vi "Rasnik.vi"() -> ()   [LabVIEW 2015]
uses:
  GlobalPath.vi
  GlobalData.vi
panel:
  out "angle D10":dbl format="%.2f"
  out "angle D9":dbl format="%.2f"
  out "angle D8":dbl format="%.2f"
  out "angle D7":dbl format="%.2f"
  out "angle D6":dbl format="%.2f"
  out "angle D5":dbl format="%.2f"
  out "angle D4":dbl format="%.2f"
  out "angle D3":dbl format="%.2f"
  out "angle D2":dbl format="%.2f"
  out "angle D1":dbl format="%.2f"
  out "Y D10":dbl format="%.2f"
  out "Y D9":dbl format="%.2f"
  out "Y D8":dbl format="%.2f"
  out "Y D7":dbl format="%.2f"
  out "Y D6":dbl format="%.2f"
  out "Y D5":dbl format="%.2f"
  out "Y D4":dbl format="%.2f"
  out "Y D3":dbl format="%.2f"
  out "Y D2":dbl format="%.2f"
  out "Y D1":dbl format="%.2f"
  out "X D10":dbl format="%.2f"
  out "X D9":dbl format="%.2f"
  out "X D8":dbl format="%.2f"
  out "X D7":dbl format="%.2f"
  out "X D6":dbl format="%.2f"
  out "X D5":dbl format="%.2f"
  out "X D4":dbl format="%.2f"
  out "X D3":dbl format="%.2f"
  out "X D2":dbl format="%.2f"
  out "X D1":dbl format="%.2f"
  out "filenames 2":string[](array[string])
  out "Latest file: 2":path
  out "angle 6":string
  out "y 6":string
  out "x 6":string
  out "filenames":string[](array[string])
  out "path":path
  in  "Done?":bool
  out "angle 10":string
  out "y 10":string
  out "x 10":string
  out "angle 9":string
  out "y 9":string
  out "x 9":string
  out "angle 8":string
  out "y 8":string
  out "x 8":string
  out "angle 7":string
  out "y 7":string
  out "x 7":string
  out "angle 5":string
  out "y 5":string
  out "x 5":string
  out "angle 4":string
  out "y 4":string
  out "x 4":string
  out "angle 3":string
  out "y 3":string
  out "x 3":string
  out "angle 2":string
  out "y 2":string
  out "x 2":string
  out "angle 1":string
  out "y 1":string
  out "x 1":string
  out "Lines":string[](array[string])
  out "Latest file:":path
  in  "Open Program":bool
  in  "c-ccd 3":bool caption="Setup the electronics for the C-CCD reading"
  in  "c-ccd":bool caption="Read the data file"
  # "Rasmask reading from PCBs on stiffback/table"
  # "Run the C-CCD reading program \n(the 10 Rasmasks are automatically read and the data saved)"
  # "Data file reading"
  # "The most recent data file created by the C-CCD program will be opened.\nOnce the \"read data file\" is clicked, the raw data and displacement should appear on the PCB schematics on the bottom."
  # "Displacement (um):"
  # "Raw Data (um):"
  # "Rasmask 1"
  # "Rasmask 2"
  # "Rasmask 1"
  # "Rasmask 2"
  # "Rasmask 3"
  # "Rasmask 4"
  # "Rasmask 3"
  # "Rasmask 4"
  # "Rasmask 6"
  # "Rasmask 5"
  # "Rasmask 6"
  # "Rasmask 5"
  # "Rasmask 7"
  # "Rasmask 8"
  # "Rasmask 7"
  # "Rasmask 8"
  # "Rasmask 9"
  # "Rasmask 10"
  # "Rasmask 9"
  # "Rasmask 10"
  # "Open the DB and load the Rarnik raw file:\nClick on the tab \"RO measurement\" and on the bottom click on \"Load Rasnik 1\" for the table and \"Load  Rasnik 2\" for the stiffback\nLoad the file that appears here --------------------------------------------------------------->\nPress \"SAve info to database\""
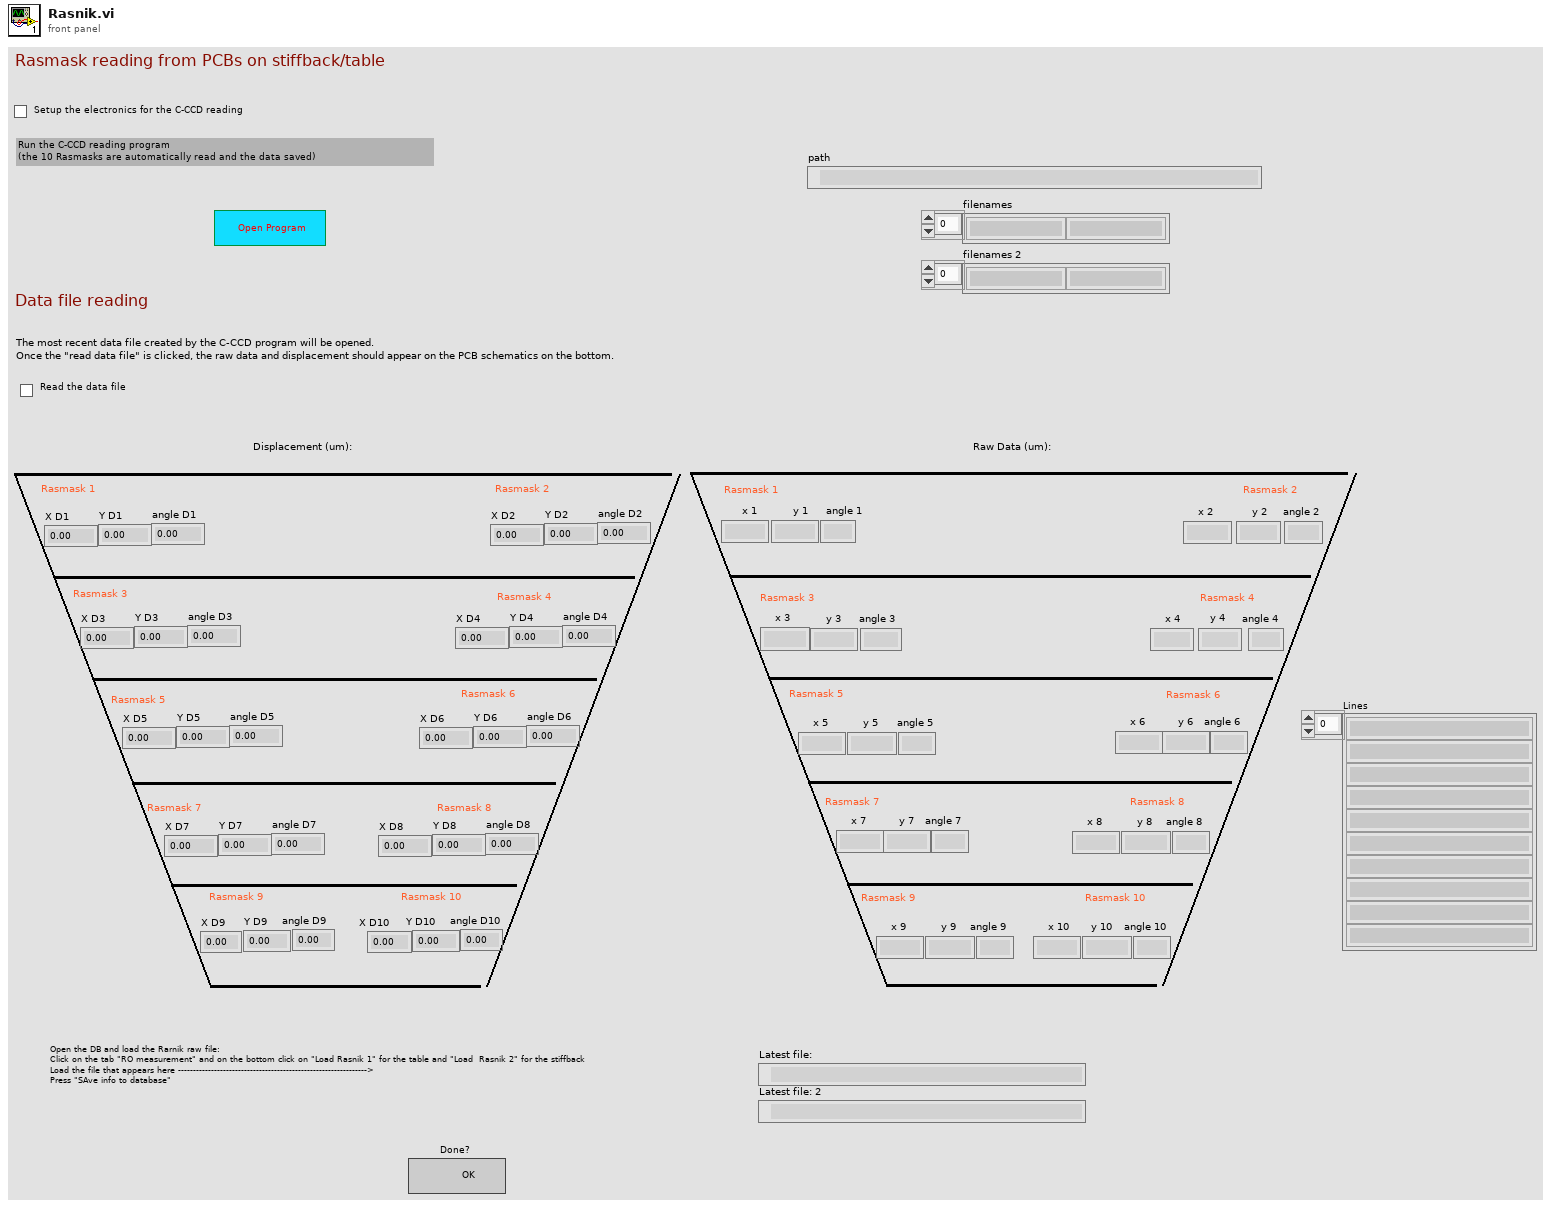
[diagram p1: front panel]
types:
  T1 = enum16{"open", "replace", "create", "open or create", "replace or create", "replace or create with confirmation"}
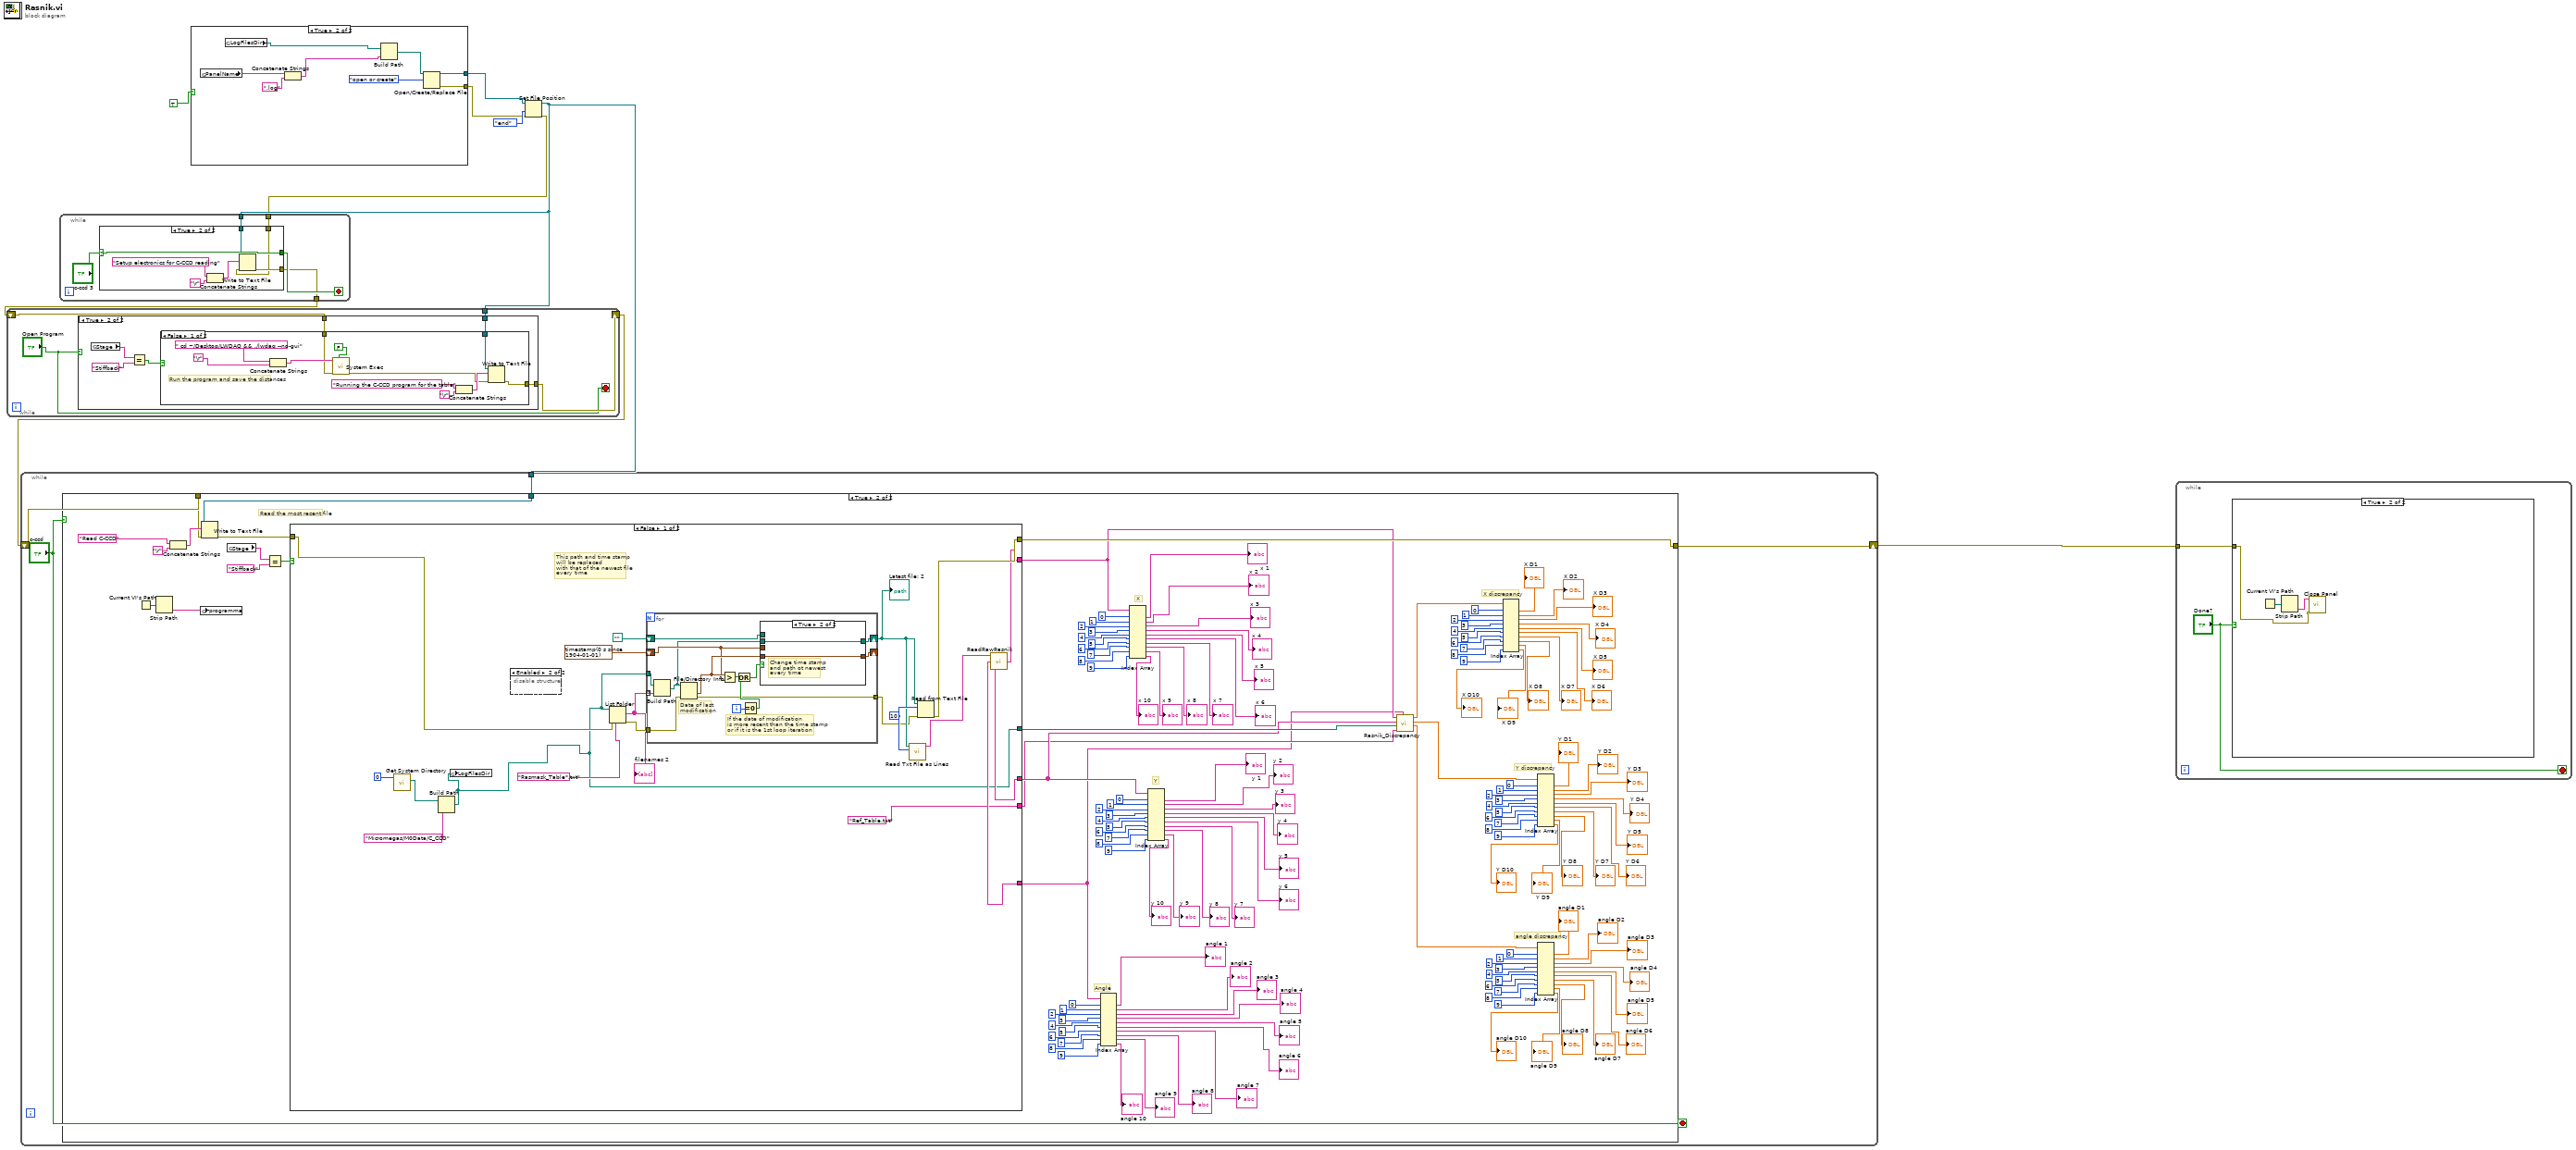
[diagram p0: block diagram]
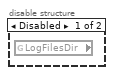
[diagram p4: hidden frame]
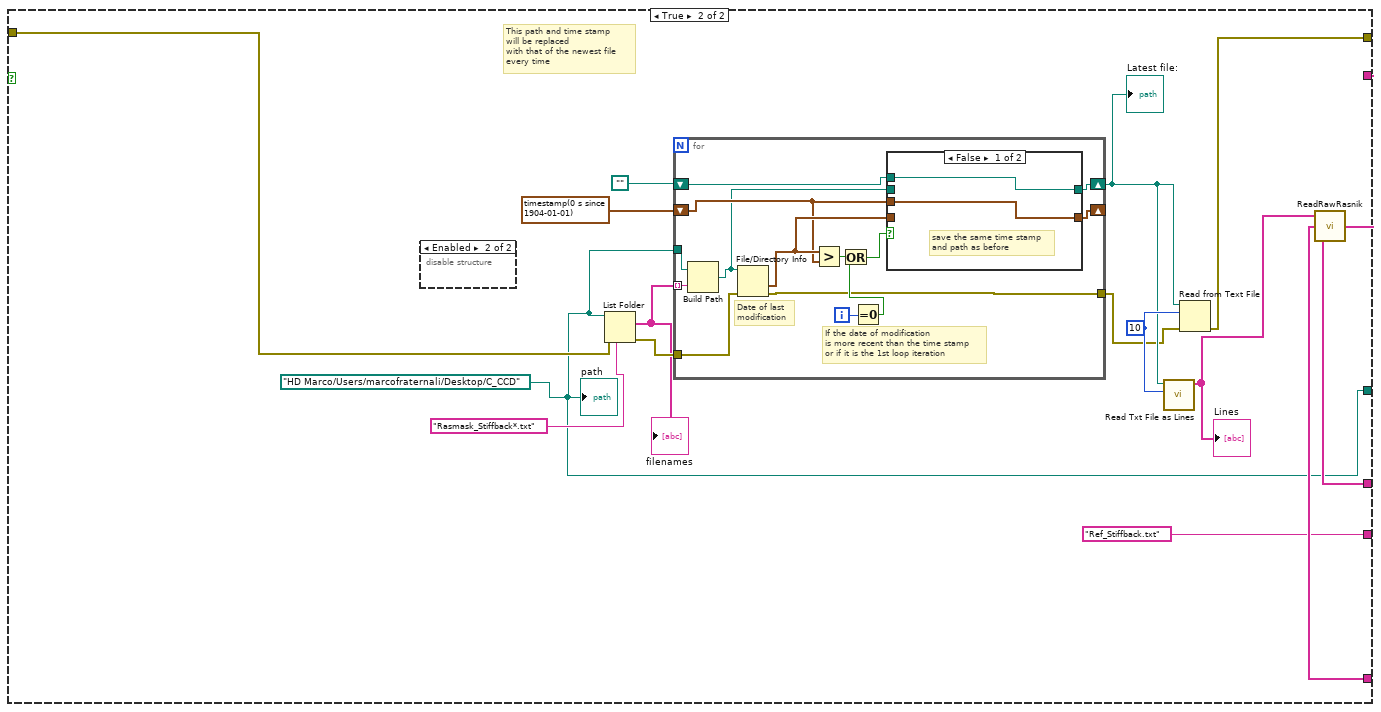
[diagram p6: hidden frame]
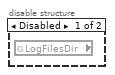
[diagram p7: hidden frame]
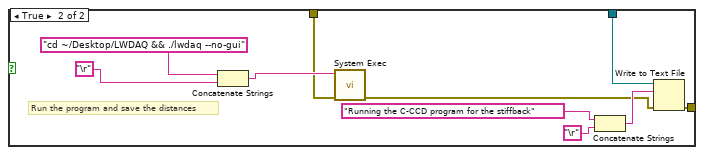
[diagram p11: hidden frame]
diagram:
  n1 = case shown="True" TRUE {
    tunnel: [_ w16] -> w3
    tunnel: [_ w15] -> w4
    frame False {
    }
    frame True {
      n2 = global read "GlobalData.vi" "PanelName"() -> (w11:string)
      n3 = global read "GlobalPath.vi" "LogFilesDir"() -> (w13:path)
      n4 = Concatenate Strings(w11, ".log") -> (w10:string)
      n5 = Build Path(base path=w13, name or relative path=w10) -> (appended path=w17:path)
      n6 = Open/Create/Replace File(file path (use dialog)=w17, operation (0:open)=T1."open or create") -> (refnum out=w16:refnum<file>, error out=w15:errorcluster)  [unwired: 4 in, 1 out]
    }
  }
  n7 = Set File Position(refnum=w3, from (0:start)=enum16{"start", "end", "current"}."end", error in=w4) -> (refnum out=w2:refnum<file>, error out=w1:errorcluster)  [unwired: 1 in]
  n8 = while {
    tunnel: w2 -> [w21]
    tunnel: [w19] -> w7
    tunnel: w1 -> [w18]
    stop <- w20 stop-if-true
    n9 = case shown="True" "c-ccd 3" {
      selector: "c-ccd 3" -> [_ w25]
      tunnel: [_ w26] -> w19
      tunnel: w21 -> [_ w23]
      tunnel: [_ w25] -> w20
      tunnel: w18 -> [_ w24]
      frame False {
      }
      frame True {
        n10 = Concatenate Strings("Setup electronics for C-CCD reading", "\r") -> (w29:string)
        n11 = Write to Text File(file (use dialog)=w23, text=w29, error in=w24) -> (error out=w26:errorcluster)  [unwired: 1 in, 2 out]
      }
    }
  }
  n12 = while {
    tunnel: w2 -> [w31]
    shift-right: [w32] -> w9
    shift-left: w7 -> [w33]
    stop <- "Open Program" stop-if-true
    n13 = case shown="True" "Open Program" {
      tunnel: w33 -> [w34 w37]
      tunnel: [w34 w36] -> w32
      tunnel: w31 -> [_ w35]
      frame False {
      }
      frame True {
        n14 = global read "GlobalData.vi" "Stage"() -> (w39:string)
        n15 = Equal?(x=w39, y="Stiffback") -> (x = y?=w38:bool)
        n16 = case shown="False" w38 {
          tunnel: w37 -> [w45 w55]
          tunnel: [w43 w53] -> w36
          tunnel: w35 -> [w42 w52]
          frame False {
            # "Run the program and save the distances"
            n17 = Concatenate Strings(" cd ~/Desktop/LWDAQ && ./lwdaq --no-gui", "\r") -> (w50:string)
            n18 = call <vilib>:"System Exec.vi"("wait until completion? (T)"=FALSE, "error in (no error)"=w45, "command line"=w50) -> ("error out"=w44:errorcluster)  [unwired: 5 in, 3 out]
            n19 = Concatenate Strings("Running the C-CCD program for the table", "\r") -> (w48:string)
            n20 = Write to Text File(file (use dialog)=w42, text=w48, error in=w44) -> (error out=w43:errorcluster)  [unwired: 1 in, 2 out]
          }
          frame True {
            # "Run the program and save the distances"
            n21 = Concatenate Strings("cd ~/Desktop/LWDAQ && ./lwdaq --no-gui", "\r") -> (w60:string)
            n22 = call <vilib>:"System Exec.vi"("error in (no error)"=w55, "command line"=w60) -> ("error out"=w54:errorcluster)  [unwired: 6 in, 3 out]
            n23 = Concatenate Strings("Running the C-CCD program for the stiffback", "\r") -> (w58:string)
            n24 = Write to Text File(file (use dialog)=w52, text=w58, error in=w54) -> (error out=w53:errorcluster)  [unwired: 1 in, 2 out]
          }
        }
      }
    }
  }
  n25 = while {
    tunnel: w2 -> [w63]
    shift-right: [w64] -> w8
    shift-left: w9 -> [w65]
    stop <- "c-ccd" stop-if-true
    n26 = case shown="True" "c-ccd" {
      tunnel: w65 -> [w66 w198]
      tunnel: [w66 w196] -> w64
      tunnel: w63 -> [_ w195]
      frame False {
      }
      frame True {
        # "angle discrepancy"
        # "Y discrepancy"
        # "X discrepancy"
        # "Angle"
        # "Y"
        # "X"
        # "Read the most recent file"
        n27 = Current VI's Path() -> (path=w199:path)
        n28 = Strip Path(path=w199) -> (name=w200:string)  [unwired: 1 out]
        n29 = Concatenate Strings("Read C-CCD", "\r") -> (w206:string)
        n30 = global write "GlobalData.vi" "programma"(w200) -> ()
        n31 = Write to Text File(file (use dialog)=w195, text=w206, error in=w198) -> (error out=w197:errorcluster)  [unwired: 1 in, 2 out]
        n32 = global read "GlobalData.vi" "Stage"() -> (w202:string)
        n33 = Equal?(x=w202, y="Stiffback") -> (x = y?=w201:bool)
        n34 = case shown="False" w201 {
          tunnel: w197 -> [w212 w255]
          tunnel: [w215 w249] -> w196
          tunnel: [w214 w248] -> w133
          tunnel: [w216 w247] -> w132
          tunnel: [w213 w246] -> w67
          tunnel: [w207 w245] -> w134
          tunnel: ["Ref_Table.txt" "Ref_Stiffback.txt"] -> w131
          frame False {
            w223 = 10
            # "This path and time stamp\nwill be replaced\nwith that of the newest file \nevery time"
            n35 = call <vilib>:"Get System Directory.vi"("system directory type"=0) -> ("system directory"=w208:path)  [unwired: 10 in]
            n36 = Build Path(base path=w208, name or relative path="Micromegas/M0Data/C_CCD") -> (appended path=w207:path)
            n37 = global write "GlobalPath.vi" "LogFilesDir"(w207) -> ()
            n38 = disable-structure shown="Enabled" {
              frame Disabled {
                n39 = global read "GlobalPath.vi" "LogFilesDir"() -> ()  [unwired: 1 out]
              }
              frame Enabled {
              }
            }
            n40 = List Folder(path=w207, pattern="Rasmask_Table*.txt", error in=w212) -> (filenames=w218:string[], error out=w221:errorcluster)  [unwired: 1 in, 2 out]
            "filenames 2" <- w218
            n41 = for {
              tunnel: w218 -> [w229] mode=indexing
              tunnel: w207 -> [w239]
              shift-right: [w234] -> _
              shift-left: timestamp(0 s since 1904-01-01) ("last mod 2") -> [w232]
              shift-right: [w233] -> w222
              shift-left: path "" -> [w230]
              tunnel: w221 -> [w227]
              tunnel: [w226] -> w220
              i -> [w237]
              # "If the date of modification\nis more recent than the time stamp\nor if it is the 1st loop iteration"
              # "Date of last\nmodification"
              n42 = Build Path(base path=w239, name or relative path=w229) -> (appended path=w228:path)
              n43 = File/Directory Info(path=w228, error in=w227) -> (last mod=w235:timestamp, error out=w226:errorcluster)  [unwired: 5 out]
              n44 = Greater?(x=w235, y=w232) -> (0:w238:bool)
              n45 = Equal To 0?(x=w237) -> (x = 0?=w236:bool)
              n46 = Or(x=w238, y=w236) -> (x .or. y?=w231:bool)
              n47 = case shown="True" w231 {
                tunnel: w232 -> [w241 _]
                tunnel: w235 -> [_ w243]
                tunnel: w228 -> [_ w242]
                tunnel: [w240 w242] -> w233
                tunnel: w230 -> [w240 _]
                tunnel: [w241 w243] -> w234
                frame False {
                  # "save the same time stamp \nand path as before"
                }
                frame True {
                  # "Change time stamp\nand path ot newest \nevery time"
                }
              }
            }
            "Latest file: 2" <- w222
            n48 = call "Read Txt File as Lines.vi"("Lines to Read"=w223, "file path (use dialog)"=w222) -> ("Lines"=w219:string[])  [unwired: 8 in, 1 out]
            n49 = Read from Text File(file (use dialog)=w222, count=w223, error in=w220) -> (error out=w215:errorcluster)  [unwired: 1 in, 3 out]
            n50 = call "ReadRawRasnik.vi"("Lines"=w219) -> ("X cluster"=w214:string[], "Y cluster"=w216:string[], "angle cluster"=w213:string[])
          }
          frame True {
            w245 = path "/HD Marco/Users/marcofraternali/Desktop/C_CCD" ("path")
            w257 = 10
            # "This path and time stamp\nwill be replaced\nwith that of the newest file \nevery time"
            n51 = disable-structure shown="Enabled" {
              frame Disabled {
                n52 = global read "GlobalPath.vi" "LogFilesDir"() -> ()  [unwired: 1 out]
              }
              frame Enabled {
              }
            }
            n53 = List Folder(path=w245, pattern="Rasmask_Stiffback*.txt", error in=w255) -> (filenames=w251:string[], error out=w254:errorcluster)  [unwired: 1 in, 2 out]
            "filenames" <- w251
            n54 = for {
              tunnel: w251 -> [w263] mode=indexing
              tunnel: w245 -> [w273]
              shift-right: [w268] -> _
              shift-left: timestamp(0 s since 1904-01-01) ("last mod 2") -> [w266]
              shift-right: [w267] -> w256
              shift-left: path "" -> [w264]
              tunnel: w254 -> [w261]
              tunnel: [w260] -> w253
              i -> [w271]
              # "If the date of modification\nis more recent than the time stamp\nor if it is the 1st loop iteration"
              # "Date of last\nmodification"
              n55 = Build Path(base path=w273, name or relative path=w263) -> (appended path=w262:path)
              n56 = File/Directory Info(path=w262, error in=w261) -> (last mod=w269:timestamp, error out=w260:errorcluster)  [unwired: 5 out]
              n57 = Greater?(x=w269, y=w266) -> (0:w272:bool)
              n58 = Equal To 0?(x=w271) -> (x = 0?=w270:bool)
              n59 = Or(x=w272, y=w270) -> (x .or. y?=w265:bool)
              n60 = case shown="False" w265 {
                tunnel: w266 -> [w275 _]
                tunnel: w269 -> [_ w277]
                tunnel: w262 -> [_ w276]
                tunnel: [w274 w276] -> w267
                tunnel: w264 -> [w274 _]
                tunnel: [w275 w277] -> w268
                frame False {
                  # "save the same time stamp \nand path as before"
                }
                frame True {
                  # "Change time stamp\nand path ot newest \nevery time"
                }
              }
            }
            "Latest file:" <- w256
            n61 = call "Read Txt File as Lines.vi"("Lines to Read"=w257, "file path (use dialog)"=w256) -> ("Lines"=w252:string[])  [unwired: 8 in, 1 out]
            "Lines" <- w252
            n62 = Read from Text File(file (use dialog)=w256, count=w257, error in=w253) -> (error out=w249:errorcluster)  [unwired: 1 in, 3 out]
            n63 = call "ReadRawRasnik.vi"("Lines"=w252) -> ("X cluster"=w248:string[], "Y cluster"=w247:string[], "angle cluster"=w246:string[])
            "path" <- w245
          }
        }
        n64 = Index Array(array=w67, index #1=0, index #2=1, index #3=2, index #4=3, index #5=4, index #6=5, index #7=6, index #8=7, index #9=8, index #10=9) -> (element #1=→"angle 1":string, element #2=→"angle 2":string, element #3=→"angle 3":string, element #4=→"angle 4":string, element #5=→"angle 5":string, element #6=→"angle 6":string, element #7=→"angle 7":string, element #8=→"angle 8":string, element #9=→"angle 9":string, element #10=→"angle 10":string)
        n65 = Index Array(array=w133, index #1=0, index #2=1, index #3=2, index #4=3, index #5=4, index #6=5, index #7=6, index #8=7, index #9=8, index #10=9) -> (element #1=→"x 1":string, element #2=→"x 2":string, element #3=→"x 3":string, element #4=→"x 4":string, element #5=→"x 5":string, element #6=→"x 6":string, element #7=→"x 7":string, element #8=→"x 8":string, element #9=→"x 9":string, element #10=→"x 10":string)
        n66 = Index Array(array=w132, index #1=0, index #2=1, index #3=2, index #4=3, index #5=4, index #6=5, index #7=6, index #8=7, index #9=8, index #10=9) -> (element #1=→"y 1":string, element #2=→"y 2":string, element #3=→"y 3":string, element #4=→"y 4":string, element #5=→"y 5":string, element #6=→"y 6":string, element #7=→"y 7":string, element #8=→"y 8":string, element #9=→"y 9":string, element #10=→"y 10":string)
        n67 = call "Rasnik_Discrepancy.vi"("angle array"=w67, "pattern"=w131, "path"=w134, "Y array"=w132, "X array"=w133) -> ("angle discrepancy"=w69:dbl[], "Y discrepancy"=w70:dbl[], "X discrepancy"=w68:dbl[])  [unwired: 4 in]
        n68 = Index Array(array=w68, index #1=0, index #2=1, index #3=2, index #4=3, index #5=4, index #6=5, index #7=6, index #8=7, index #9=8, index #10=9) -> (element #1=→"X D1":dbl, element #2=→"X D2":dbl, element #3=→"X D3":dbl, element #4=→"X D4":dbl, element #5=→"X D5":dbl, element #6=→"X D6":dbl, element #7=→"X D7":dbl, element #8=→"X D8":dbl, element #9=→"X D9":dbl, element #10=→"X D10":dbl)
        n69 = Index Array(array=w70, index #1=0, index #2=1, index #3=2, index #4=3, index #5=4, index #6=5, index #7=6, index #8=7, index #9=8, index #10=9) -> (element #1=→"Y D1":dbl, element #2=→"Y D2":dbl, element #3=→"Y D3":dbl, element #4=→"Y D4":dbl, element #5=→"Y D5":dbl, element #6=→"Y D6":dbl, element #7=→"Y D7":dbl, element #8=→"Y D8":dbl, element #9=→"Y D9":dbl, element #10=→"Y D10":dbl)
        n70 = Index Array(array=w69, index #1=0, index #2=1, index #3=2, index #4=3, index #5=4, index #6=5, index #7=6, index #8=7, index #9=8, index #10=9) -> (element #1=→"angle D1":dbl, element #2=→"angle D2":dbl, element #3=→"angle D3":dbl, element #4=→"angle D4":dbl, element #5=→"angle D5":dbl, element #6=→"angle D6":dbl, element #7=→"angle D7":dbl, element #8=→"angle D8":dbl, element #9=→"angle D9":dbl, element #10=→"angle D10":dbl)
      }
    }
  }
  n71 = while {
    tunnel: w8 -> [w279]
    stop <- "Done?" stop-if-true
    n72 = case shown="True" "Done?" {
      tunnel: w279 -> [_ w280]
      frame False {
      }
      frame True {
        n73 = Current VI's Path() -> (path=w281:path)
        n74 = Strip Path(path=w281) -> (name=w282:string)  [unwired: 1 out]
        n75 = call <vilib>:"Close Panel.vi"("error in (no error)"=w280, "VI name"=w282) -> ()  [unwired: 9 in, 1 out]
      }
    }
  }
